vi "删除启动项.vi"(8 "error in (no error)":errorcluster caption="错误输入（无错误）", 11 "启动文件路径":path) -> (0 "error out":errorcluster caption="错误输出", 3 "删除标记":bool)   [LabVIEW 2016, in "中水三立SQL数据传输.lvlib"]
uses:
  <vilib>/registry/registry.llb/Registry RtKey.ctl
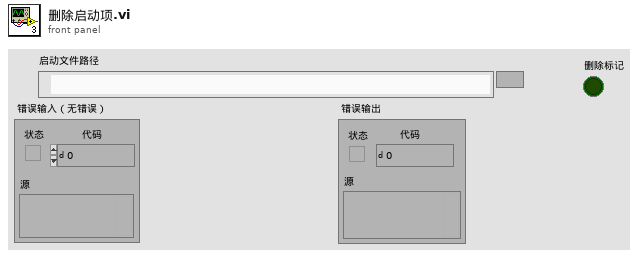
[diagram p1: front panel]
types:
  T1 = typedef "Registry RtKey.ctl" = enum32{"HKEY_CLASSES_ROOT", "HKEY_CURRENT_USER", "HKEY_LOCAL_MACHINE", "HKEY_USERS", "HKEY_PERFORMANCE_DATA", "HKEY_CURRENT_CONFIG", "HKEY_DYN_DATA"}
  T2 = typedef "Registry refnum.ctl" = refnum<k1>
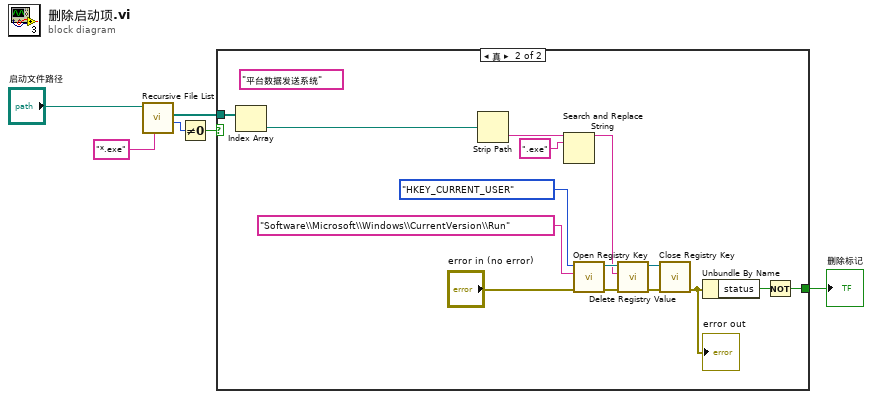
[diagram p0: block diagram]
diagram:
  n1 = call <vilib>:"Recursive File List.vi"("pattern"="*.exe", "Folder Path"="启动文件路径") -> ("Number of Files"=w3:i32, "All Files in Dir"=w4:path[])  [unwired: 5 in, 3 out]
  n2 = Not Equal To 0?(x=w3) -> (x != 0?=w2:bool)
  n3 = case shown="真" w2 {
    tunnel: w4 -> [_ w21]
    tunnel: [_ w8] -> w1
    frame False {
    }
    frame True {
      (unwired) "平台数据发送系统" ("value")
      n4 = Index Array(array=w21) -> (element=w20:path)  [unwired: 1 in]
      n5 = Strip Path(path=w20) -> (name=w19:string)  [unwired: 1 out]
      n6 = Search and Replace String(input string=w19, search string=".exe" ("搜索字符串")) -> (result string=w7:string)  [unwired: 6 in, 3 out]
      n7 = call <vilib>:"Open Registry Key.vi"("error in (no error)"="error in (no error)", "subkey"="Software\\Microsoft\\Windows\\CurrentVersion\\Run", "root key (HKEY_LOCAL_MACHINE)"=Registry_RtKey."HKEY_CURRENT_USER") -> ("error out"=w13:errorcluster, "refnum out"=w15:T2)  [unwired: 7 in]
      n8 = call <vilib>:"Delete Registry Value.vi"("error in (no error)"=w13, "value"=w7, "refnum"=w15) -> ("error out"=w12:errorcluster, "refnum out"=w14:T2)  [unwired: 7 in]
      n9 = call <vilib>:"Close Registry Key.vi"("error in (no error)"=w12, "refnum"=w14) -> ("error out"=w10:errorcluster)  [unwired: 5 in]
      "error out" <- w10
      n10 = Unbundle By Name(w10) -> ("status"=w9:bool)
      n11 = Not(x=w9) -> (.not. x?=w8:bool)
    }
  }
  "删除标记" <- w1
